vi "EstimateGCost.vi"(9 "Nó pai":dbl[](array[numeric]), 10 "Nó atual":dbl[](array[numeric])=[2.0, 1.0, 3.0, 0.0, 0.0, 0.0], 11 "GridParameter":dbl) -> (2 "G_Cost":dbl)   [LabVIEW 2016]
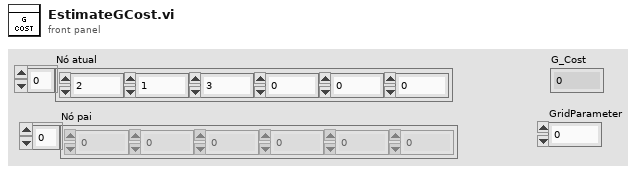
[diagram p1: front panel]
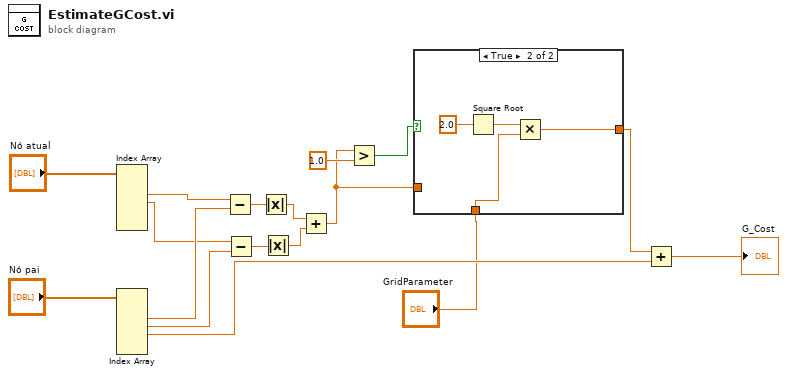
[diagram p0: block diagram]
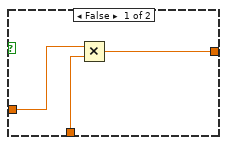
[diagram p2: hidden frame]
diagram:
  n1 = Index Array(array="Nó atual") -> (element #2=w14:dbl, element #3=w11:dbl)  [unwired: 6 in, 4 out]
  n2 = Index Array(array="Nó pai") -> (element #2=w13:dbl, element #3=w10:dbl, element #4=w15:dbl)  [unwired: 6 in, 3 out]
  n3 = Subtract(x=w14, y=w13) -> (x-y=w12:dbl)
  n4 = Subtract(x=w11, y=w10) -> (x-y=w9:dbl)
  n5 = Absolute Value(x=w12) -> (abs(x)=w7:dbl)
  n6 = Absolute Value(x=w9) -> (abs(x)=w8:dbl)
  n7 = Add(x=w7, y=w8) -> (x+y=w3:dbl)
  n8 = Greater?(x=w3, y=1.0) -> (0:w4:bool)
  n9 = case shown="True" w4 {
    tunnel: w3 -> [w20 _]
    tunnel: "GridParameter" -> [w19 w22]
    tunnel: [w18 w21] -> w1
    frame False {
      n10 = Multiply(x=w20, y=w19) -> (x*y=w18:dbl)
    }
    frame True {
      n11 = Square Root(x=2.0) -> (sqrt(x)=w23:dbl)
      n12 = Multiply(x=w23, y=w22) -> (x*y=w21:dbl)
    }
  }
  n13 = Add(x=w1, y=w15) -> (x+y=→"G_Cost":dbl)
